vi "Get Port Config.vi"(8 "error in (no error)":errorcluster, 11 "Serial Client in":refnum<class "Serial Client.lvclass">) -> (0 "error out":errorcluster, 2 "Port Config":T1={"Baud (115200)"=115200, "Data Bits (8)"=8, "Stop Bits (1)"=10, "Flow Control"=0, "Use LineTerm?"=FALSE, "LineTerm (\\n)"="\n", "Timeout ms (10000)"=10000, "Parity (None)"=enum."None"} {"Flow Control" items=["None", "XON/XOFF", "RTS/CTS", "XON/XOFF & RTS/CTS", "DTR/DSR", "XON/XOFF & DTR/DSR"]; "Stop Bits (1)" items=["1.0"=10, "1.5"=15, "2.0"=20]}, 3 "Serial Client out":refnum<class "Serial Client.lvclass">)   [LabVIEW 2020, in "Stream-Serial.lvlib" / "Serial Client.lvclass"]
doc: "Returns the currently set port configuration."
uses:
  Serial Client.lvclass
  Port Config.ctl
  Stop Bits.ctl
  Flow Control.ctl
  Parity.ctl
  Serial Client.lvclass/Serial Client.ctl
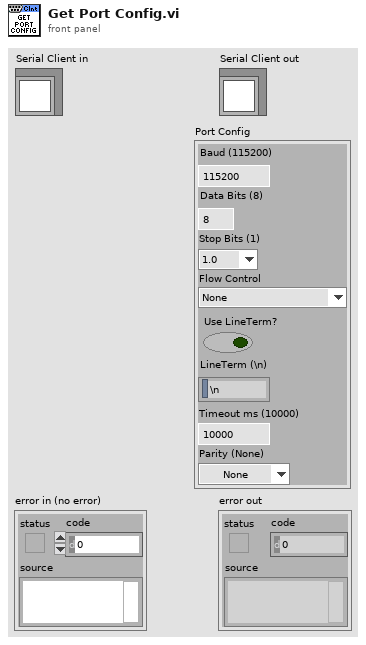
[diagram p1: front panel]
types:
  T1 = typedef "Stream-Serial.lvlib/Serial Client.lvclass/Port Config.ctl" = cluster{"Baud (115200)":u32, "Data Bits (8)":u8, "Stop Bits (1)":T2, "Flow Control":T3, "Use LineTerm?":bool, "LineTerm (\\n)":string, "Timeout ms (10000)":i32, "Parity (None)":T4}
  T2 = typedef "Stream-Serial.lvlib/Serial Client.lvclass/Stop Bits.ctl" = u16
  T3 = typedef "Stream-Serial.lvlib/Serial Client.lvclass/Flow Control.ctl" = u16
  T4 = typedef "Stream-Serial.lvlib/Serial Client.lvclass/Parity.ctl" = enum16{"None", "Odd", "Even", "Mark", "Space"}
  T5 = typedef "Stream-Serial.lvlib/Serial Client.lvclass/Ref Data.ctl" = cluster{"Stream":refnum<class "Serial Stream.lvclass">, "Client Loop":refnum<vi>, "Port Config":T1, "VISA Resource":refnum<visa-resource-name>}
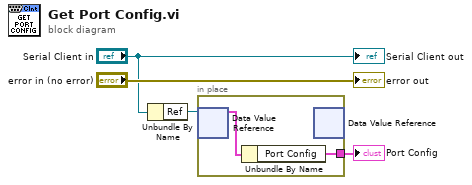
[diagram p0: block diagram]
diagram:
  n1 = Unbundle By Name("Serial Client in") -> ("Ref"=w3:refnum<data-value>)
  n2 = in-place {
    in-place-border: [w5] -> w1
    n3 = in-place-dvr #1(w3) -> (w6:T5)  [unwired: 1 out]
    n4 = Unbundle By Name(w6) -> ("Port Config"=w5:T1)
    n5 = in-place-dvr #1() -> ()  [unwired: 1 in, 2 out]
  }
  "Port Config" <- w1
  "error out" <- "error in (no error)"
  "Serial Client out" <- "Serial Client in"
